vi "TIP STRIP DEMO.vi"() -> ()   [LabVIEW 2020]
panel:
  out "Waveform Chart":dbl(graph)
  in  "Numeric without Tip Strip":dbl
  out "String":string="Tip strips appear on mouseover and disappear on mouse out or on mouse click.\n\nRegistering all FP controls might be a good way to check if all FP objects are documented.\n"
  in  "Numeric with long tip strip":dbl
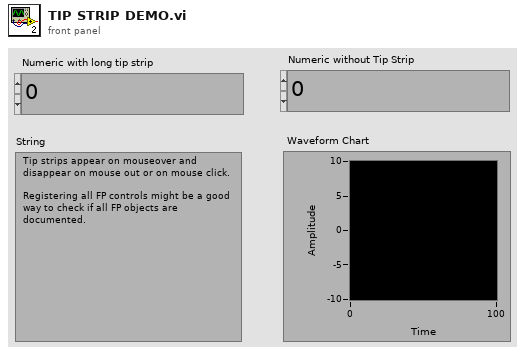
[diagram p1: front panel]
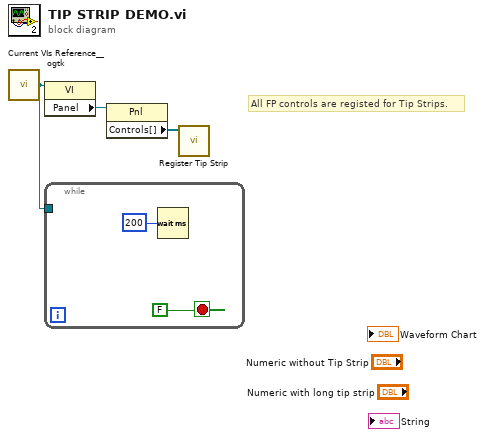
[diagram p0: block diagram]
diagram:
  # "All FP controls are registed for Tip Strips."
  n1 = call <userlib>:"Current VIs Reference__ogtk.vi"() -> ("Current VI's reference"=w3:refnum<vi>)  [unwired: 5 in]
  n2 = property class="VI"(reference=w3) -> ("Panel"=w2:refnum<vi>)  [unwired: 1 in, 2 out]
  n3 = while {
    tunnel: w3 -> [_]
    stop <- FALSE stop-if-true
    n4 = Wait (ms)(milliseconds to wait=u32 200) -> ()  [unwired: 1 out]
  }
  n5 = property class="Pnl"(reference=w2) -> ("Controls[]"=w1:refnum<vi>[])  [unwired: 1 in, 2 out]
  n6 = call "Register Tip Strip.vi"("Controls[]"=w1) -> ()  [unwired: 10 in, 1 out]
